vi "set up imaq aquisition.vi"(8 "error in (no error)":errorcluster, 9 "ROI":T2, 10 "use roi":bool, 11 "Interface Name":string="img0") -> (0 "error out":errorcluster, 1 "camera image is 8 bit":bool, 2 "camera image":T1, 3 "IMAQ Session Out":refnum<k11>)   [LabVIEW 2013]
uses:
  <vilib>/vision/Image Controls.llb/IMAQ Image.ctl
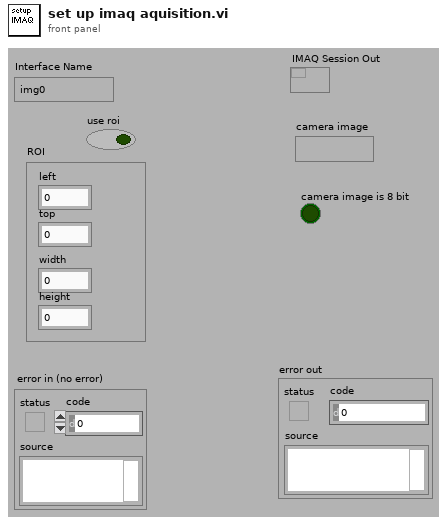
[diagram p1: front panel]
types:
  T1 = typedef "IMAQ Image.ctl" = refnum<image>
  T2 = cluster{"left":u16, "top":u16, "width":u16, "height":u16}
  T3 = typedef "Image Type" = u32
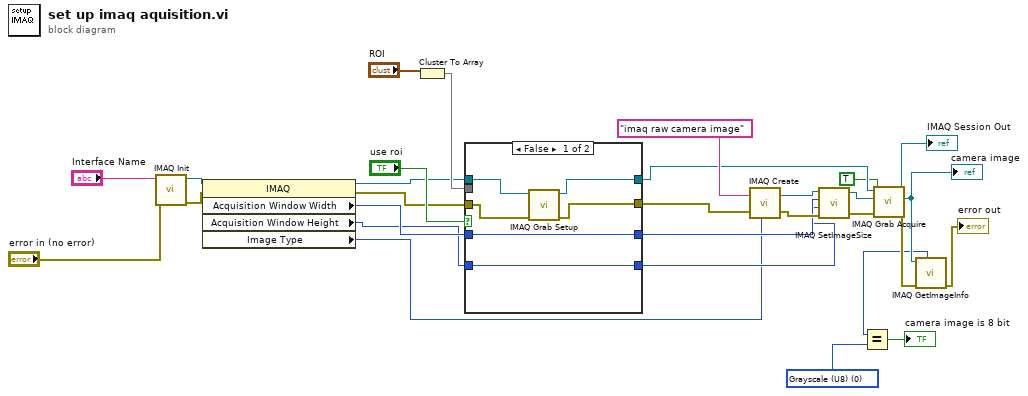
[diagram p0: block diagram]
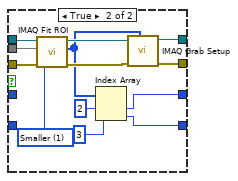
[diagram p2: hidden frame]
diagram:
  w11 = u32 0 items=["Grayscale (U8)", "Grayscale (I16)", "Grayscale (SGL)", "Complex (CSG)", "RGB (U32)", "HSL (U32)", "RGB (U64)"] ("Image Parameters : Image Type")
  n1 = call <vilib>:"IMAQ Init.vi"("error in (no error)"="error in (no error)", "Interface Name"="Interface Name") -> ("error out"=w27:errorcluster, "IMAQ Session Out"=w28:refnum<k11>)  [unwired: 8 in]
  n2 = property class="IMAQ"(reference=w28, error in=w27) -> (reference out=w22:refnum<k11>, error out=w23:errorcluster, "Acquisition Window Width"=w16:u32, "Acquisition Window Height"=w15:u32, "Image Type"=w12:u32)
  n3 = Cluster To Array(cluster="ROI") -> (array=w24:u16[])
  n4 = case shown="False" "use roi" {
    tunnel: w24 -> [_ w47]
    tunnel: w23 -> [w33 w46]
    tunnel: w22 -> [w35 w44]
    tunnel: [w34 w42] -> w7
    tunnel: [w32 w41] -> w20
    tunnel: w16 -> [w31 _]
    tunnel: w15 -> [w30 _]
    tunnel: [w31 w37] -> w14
    tunnel: [w30 w36] -> w13
    frame False {
      n5 = call <vilib>:"IMAQ Grab Setup.vi"("error in (no error)"=w33, "IMAQ Session In"=w35) -> ("error out"=w32:errorcluster, "IMAQ Session Out"=w34:refnum<k11>)  [unwired: 8 in]
    }
    frame True {
      w48 = u32 1 items=["Larger", "Smaller"] ("Fit Mode")
      n6 = call <vilib>:"IMAQ Fit ROI.vi"("error in (no error)"=w46, "Fit Mode"=w48, "Region of Interest In"=w47, "IMAQ Session In"=w44) -> ("error out"=w45:errorcluster, "Region of Interest Out"=w40:i32[], "IMAQ Session Out"=w43:refnum<k11>)  [unwired: 1 in]
      n7 = Index Array(array=w40, index #1=2 ("index"), index #2=3 ("index")) -> (element #1=w37:i32, element #2=w36:i32)
      n8 = call <vilib>:"IMAQ Grab Setup.vi"("Region of Interest"=w40, "error in (no error)"=w45, "IMAQ Session In"=w43) -> ("error out"=w41:errorcluster, "IMAQ Session Out"=w42:refnum<k11>)  [unwired: 7 in]
    }
  }
  n9 = call "IMAQ Create"("Image Name"="imaq raw camera image", "Image Type"=w12, "error in (no error)"=w20) -> ("New Image"=w17:T1, "error out"=w18:errorcluster)  [unwired: 2 in]
  n10 = call "IMAQ SetImageSize"("error in (no error)"=w18, "Y Resolution"=w13, "X Resolution"=w14, "Image"=w17) -> ("error out"=w9:errorcluster, "Image Out"=w8:T1)  [unwired: 1 in]
  n11 = call <vilib>:"IMAQ Grab Acquire.vi"("error in (no error)"=w9, "Immediate?"=TRUE, "Image In"=w8, "IMAQ Session In"=w7) -> ("error out"=w4:errorcluster, "Image Out"=w5:T1, "IMAQ Session Out"=→"IMAQ Session Out":refnum<k11>)  [unwired: 4 in, 1 out]
  "camera image" <- w5
  n12 = call "IMAQ GetImageInfo"("error in (no error)"=w4, "Image"=w5) -> ("error out"=→"error out":errorcluster, "Image Type"=w2:T3)  [unwired: 2 in, 6 out]
  n13 = Equal?(x=w2, y=w11) -> (x = y?=→"camera image is 8 bit":bool)
